vi "group Sync Read.vi"(7 "data_length":u16, 8 "error in (no error)":errorcluster, 9 "start_address":u16, 10 "protocol_version":i32, 11 "port_num":i32) -> (0 "error out":errorcluster, 3 "function return":i32)   [LabVIEW 2018, in "labview.lvlib"]
doc: "WINDECLSPEC int groupSyncRead (int port_num, int protocol_version, uint16_t start_address, uint16_t data_length);"
uses:
  labview.lvlib
  dxl_x86_c.dll
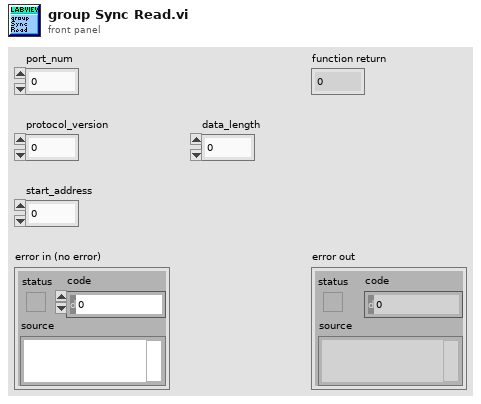
[diagram p1: front panel]
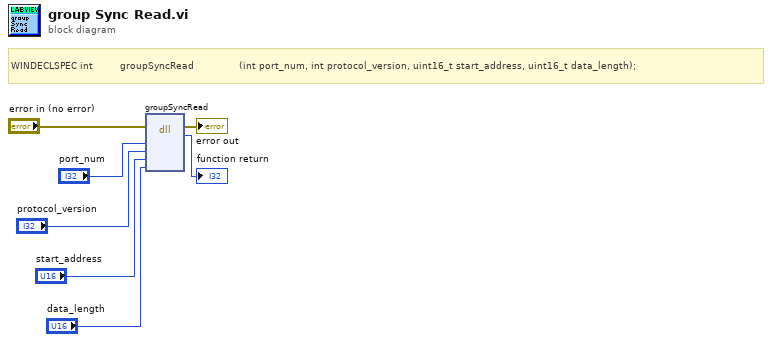
[diagram p0: block diagram]
diagram:
  # "WINDECLSPEC int         groupSyncRead               (int port_num, int protocol_version, uint16_t start_address, uint16_t data_length);"
  n1 = dll-call lib="C:/Users/joaos/OneDrive/Documents/[PhD]/Project Omnidirectional Vehicle/Vanes/LabView_code/joaoandthethreestands/DynamixelSDK-3.7.31/labview/new_compilation/dxl_x86_c.*" fn="groupSyncRead"(error in="error in (no error)", "port_num"="port_num", "protocol_version"="protocol_version", "start_address"="start_address", "data_length"="data_length") -> (error out=→"error out":errorcluster, →"function return":i32)  [unwired: 6 in, 1 out]
